vi "Tabulate_Plotted_data.vi"(3 "Data":string[][](array[string]), 4 "Channel Names":string[](array[string]), 5 "Channels to Tabulate":i32[](listbox)) -> (0 "spreadsheet string":string, 1 "Channel Values":string[][](array[string]), 2 "Channel Names":string[](array[string]))   [LabVIEW 2010]
uses:
  Results_plotter_Global.vi
panel:
  out "Table":string[][](table)
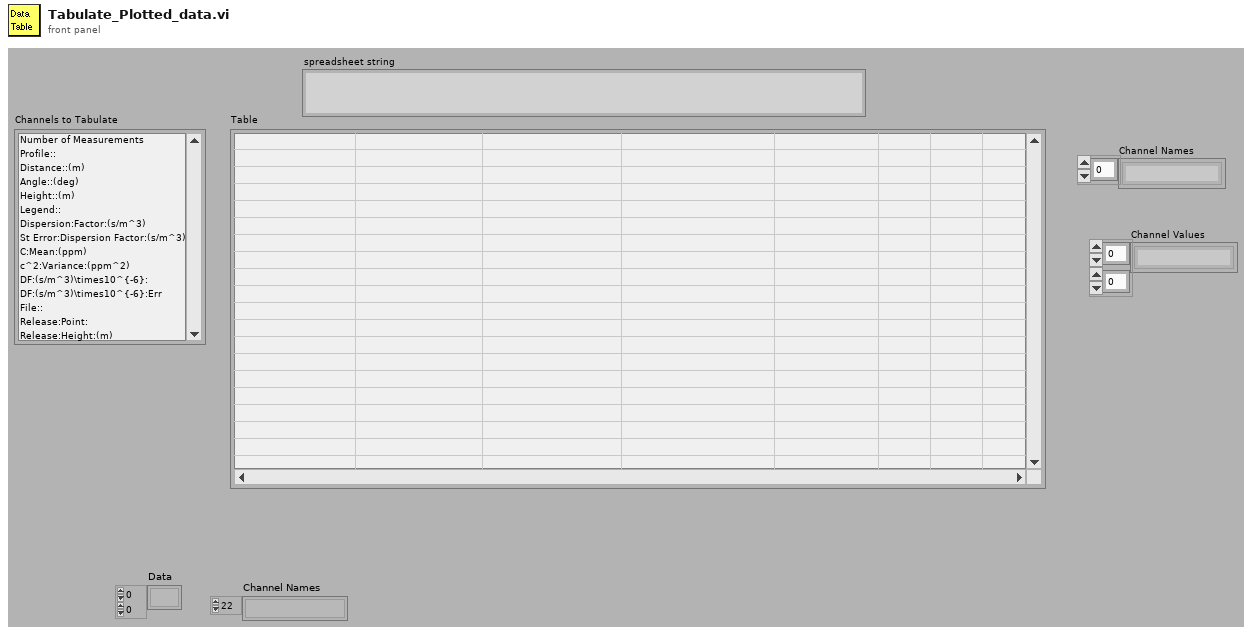
[diagram p1: front panel]
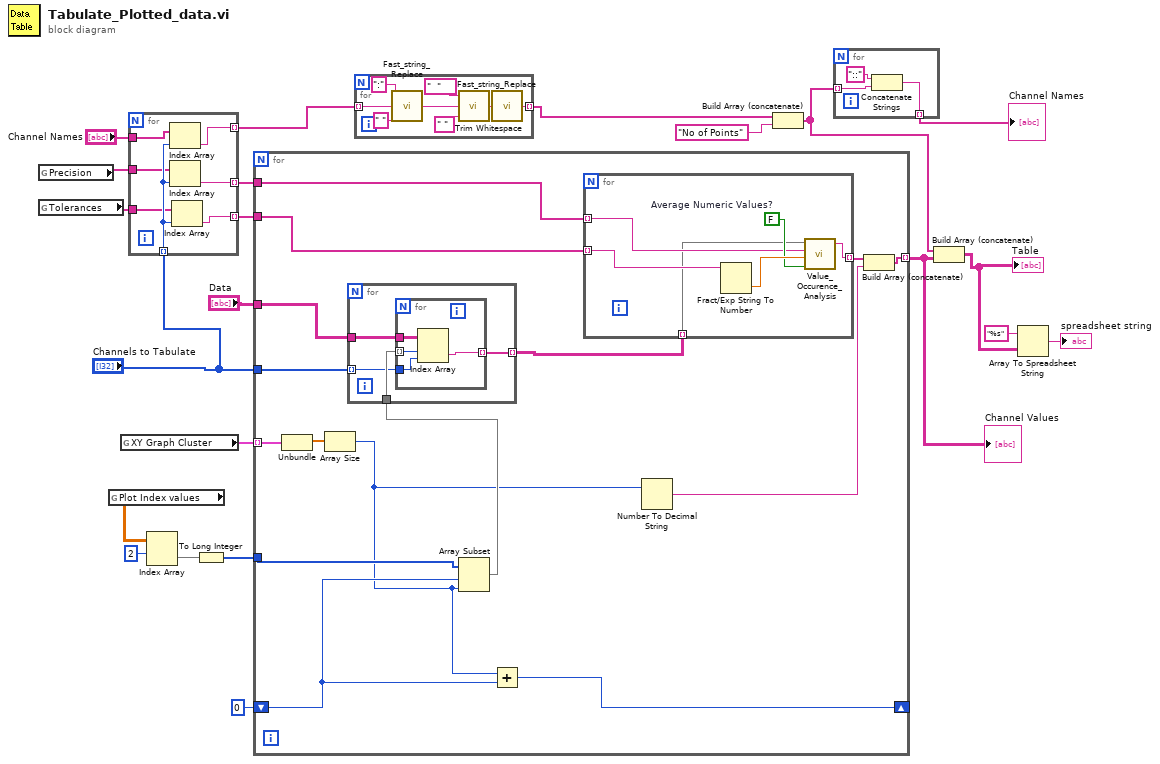
[diagram p0: block diagram]
diagram:
  n1 = global read "Results_plotter_Global.vi" "Precision"() -> (w14:string[])
  n2 = global read "Results_plotter_Global.vi" "Tolerances"() -> (w13:string[])
  n3 = global read "Results_plotter_Global.vi" "Plot Index values"() -> (w20:dbl[][])
  n4 = global read "Results_plotter_Global.vi" "XY Graph Cluster"() -> (w22:cluster{dbl[], dbl[]}[])
  n5 = for {
    tunnel: "Channels to Tabulate" -> [w29] mode=indexing
    tunnel: "Channel Names" -> [w28]
    tunnel: w14 -> [w27]
    tunnel: w13 -> [w26]
    tunnel: [w25] -> w12 mode=indexing
    tunnel: [w24] -> w11 mode=indexing
    tunnel: [w23] -> w4 mode=indexing
    n6 = Index Array(array=w28, index=w29) -> (element=w23:string)
    n7 = Index Array(array=w27, index=w29) -> (element=w25:string)
    n8 = Index Array(array=w26, index=w29) -> (element=w24:string)
  }
  n9 = Index Array(array=w20, index (row)=2) -> (element=w21:dbl[])  [unwired: 1 in]
  n10 = To Long Integer(number=w21) -> (32bit integer=w18:i32[])
  n11 = for {
    tunnel: w22 -> [w43] mode=indexing
    shift-right: [w40] -> _
    shift-left: 0 -> [w41]
    tunnel: w18 -> [w42]
    tunnel: "Data" -> [w38]
    tunnel: "Channels to Tabulate" -> [w37]
    tunnel: w12 -> [w36]
    tunnel: w11 -> [w35]
    tunnel: [w32] -> w10 mode=indexing
    n12 = Unbundle(w43) -> (w44:dbl[])  [unwired: 1 out]
    n13 = Array Size(array=w44) -> (size(s)=w31:i32)
    n14 = Array Subset(array=w42, index=w41, length=w31) -> (w39:i32[])
    n15 = for {
      tunnel: w39 -> [w48]
      tunnel: w38 -> [w47]
      tunnel: w37 -> [w46] mode=indexing
      tunnel: [w45] -> w34 mode=indexing
      n16 = for {
        tunnel: w48 -> [w52] mode=indexing
        tunnel: w47 -> [w51]
        tunnel: w46 -> [w50]
        tunnel: [w49] -> w45 mode=indexing
        n17 = Index Array(array=w51, index (row)=w52, index (col)=w50) -> (element=w49:string)
      }
    }
    n18 = Add(x=w31, y=w41) -> (x+y=w40:i32)
    n19 = for {
      tunnel: w36 -> [w56] mode=indexing
      tunnel: w35 -> [w55] mode=indexing
      tunnel: [w54] -> w33 mode=indexing
      tunnel: w34 -> [w53] mode=indexing
      w57 = FALSE  # Average Numeric Values?
      n20 = Fract/Exp String To Number(string=w55) -> (number=w58:dbl)  [unwired: 4 out]
      n21 = call "Value_Occurence_Analysis.vi"("Average Numeric Values?"=w57, "Tolerance"=w58, "Precision (3)"=w56, "String Array"=w53) -> ("Output String"=w54:string)  [unwired: 2 out]
    }
    n22 = Number To Decimal String(number=w31) -> (decimal integer string=w30:string)  [unwired: 1 out]
    n23 = Build Array (concatenate)(w33, w30) -> (w32:string[])
  }
  "Channel Values" <- w10
  n24 = for {
    tunnel: w4 -> [w66] mode=indexing
    tunnel: [w63] -> w3 mode=indexing
    n25 = call "Fast_string_Replace.vi"("Replace match with:"=" ", "Input String"=w66, "regular expression"=":") -> ("Output String"=w62:string)  [unwired: 2 out]
    n26 = call "Fast_string_Replace.vi"("Replace match with:"=" ", "Input String"=w62, "regular expression"="  ") -> ("Output String"=w61:string)  [unwired: 2 out]
    n27 = call <vilib>:"Trim Whitespace.vi"("string"=w61) -> ("trimmed string"=w63:string)  [unwired: 1 in]
  }
  n28 = Build Array (concatenate)(w3, "No of Points") -> (w1:string[])
  n29 = for {
    tunnel: w1 -> [w68] mode=indexing
    tunnel: [w67] -> w2 mode=indexing
    n30 = Concatenate Strings("::" ("regular expression"), w68) -> (w67:string)
  }
  "Channel Names" <- w2
  n31 = Build Array (concatenate)(w1, w10) -> (w8:string[][])
  "Table" <- w8
  n32 = Array To Spreadsheet String(array=w8, 3:"%s" ("format string")) -> (spreadsheet string=→"spreadsheet string":string)  [unwired: 1 out]
